vi "Write ZYState.vi"(7 "OPC UA AI list":string[](array[string]), 8 "error in (no error)":errorcluster, 10 "HE_state":T1 {"Y"."Y_Set" format="%.2f"; "Y"."SP" step=0.01 format="%.2f"; "Y"."Y" format="%.2f"; "Y"."PV" step=0.01 format="%.2f"; "Y"."SP_Set" step=0.01 format="%.2f"}, 11 "OPC UA server refnum in":T12) -> (0 "error out":errorcluster, 3 "OPC UA server refnum out":T12)   [LabVIEW 2019, in "OPC addons.lvlib"]
uses:
  OPC addons.lvlib
  <vilib>/OPCUA/controls/OPC UA Server Refnum.ctl
  Heating/ctl/ZYs_state_short.ctl
  Heating/ctl/ZY_state_short.ctl
  Heating/ctl/Z.ctl
  Heating/ctl/Z_source.ctl
  Heating/ctl/Z_State.ctl
  Heating/ctl/ZM_State.ctl
  Heating/ctl/Y_short.ctl
  Heating/ctl/Y_source.ctl
  Heating/ctl/Y_state.ctl
  Inputs/Ctl/Parameter State short.ctl
  Alarms/Ctl/ALR_Status_short.ctl
  Heating/ctl/ZY_state_OPC.ctl
  <vilib>/OPCUA/controls/Write Status.ctl
  <vilib>/OPCUA/server/Write Variant.vi
  <vilib>/OPCUA/NI OPC UA Server.lvlib
  Heating/Heating.lvlib
  Inputs/Inputs.lvlib
  Alarms/Alarms.lvlib
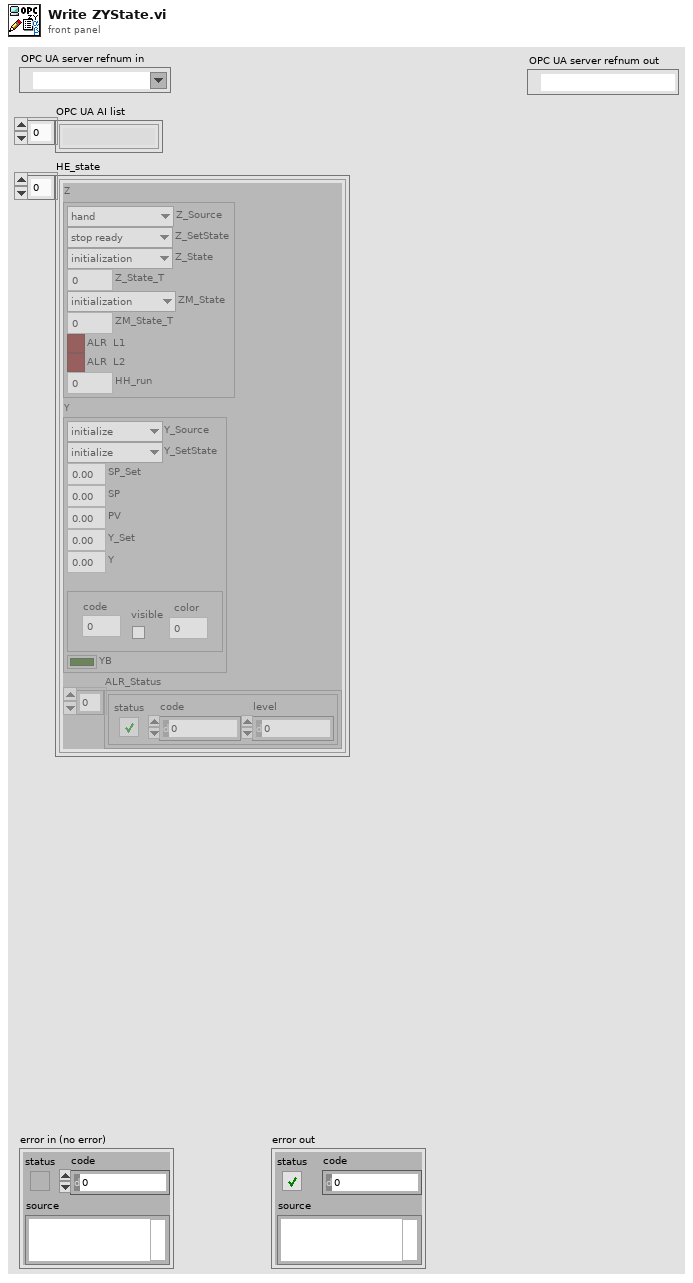
[diagram p1: front panel]
types:
  T1 = typedef "Heating.lvlib/ZYs_state_short.ctl" = T2[]
  T2 = typedef "Heating.lvlib/ZY_state_short.ctl" = cluster{"Z":T3, "Y":T7, "ALR_Status":T11[]}
  T3 = typedef "Heating.lvlib/Z.ctl" = cluster{"Z_Source":T4, "Z_SetState":T5, "Z_State":T5, "Z_State_T":u32, "ZM_State":T6, "ZM_State_T":u32, "ALR  L1":bool, "ALR  L2":bool, "HH_run":u64}
  T4 = typedef "Heating.lvlib/Z_source.ctl" = enum8{"initialize", "local disabled", "local hand", "hand", "auto", "dist"}
  T5 = typedef "Heating.lvlib/Z_State.ctl" = enum8{"initialization", "alarm", "disabled", "not ready", "stop ready", "reserv", "switched off", "reserv2", "switched on", "check", "on min", "decrease out", "on", "increase out", "on max"}
  T6 = typedef "Heating.lvlib/ZM_State.ctl" = enum8{"initialization", "stop", "start_cmd", "contactor_on_cmd", "heating", "on", "stop_cmd", "power_down", "contactor_off_cmd", "cooling", "restart_delay"}
  T7 = typedef "Heating.lvlib/Y_short.ctl" = cluster{"Y_Source":T8, "Y_SetState":T9, "SP_Set":dbl, "SP":dbl, "PV":dbl, "Y_Set":dbl, "Y":dbl, "Y_State":T10, "YB":bool}
  T8 = typedef "Heating.lvlib/Y_source.ctl" = enum8{"initialize", "local disabled", "local hand", "hand", "auto", "dist"}
  T9 = typedef "Heating.lvlib/Y_state.ctl" = enum8{"initialize", "alarm", "min", "stop", "hand", "auto", "max"}
  T10 = typedef "Inputs.lvlib/Parameter State short.ctl" = cluster{"code":i32, "visible":bool, "color":u32}
  T11 = typedef "Alarms.lvlib/ALR_Status_short.ctl" = cluster{"status":bool, "code":i32, "level":i32}
  T12 = typedef "OPC UA Server Refnum.ctl" = refnum<k21>
  T13 = typedef "Heating.lvlib/ZY_state_OPC.ctl" = cluster{"Z":cluster{"Z_Source":u8, "Z_SetState":u8, "Z_State":u8, "Z_State_T":u32, "ZM_State":u8, "ZM_State_T":u32, "ALR  L1":bool, "ALR  L2":bool, "HH_run":i32}, "Y":cluster{"Y_Source":u8, "Y_SetState":u8, "SP_Set":dbl, "SP":dbl, "PV":dbl, "Y_Set":dbl, "Y":dbl, "Y_State":cluster{"code":i32, "visible":bool, "color":u32}, "YB":bool}, "ALR_Status":cluster{"status":bool, "code":i32, "level":i32}[]}
  T14 = typedef "Write Status.ctl" = u32
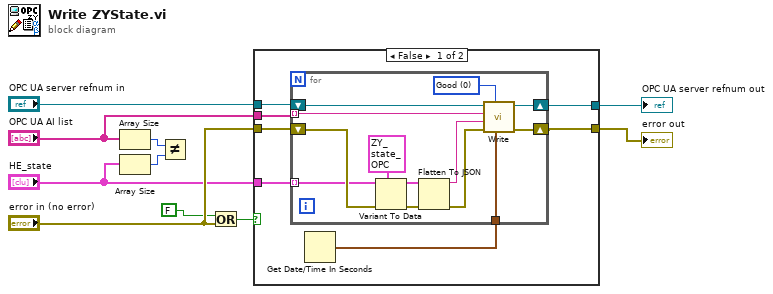
[diagram p0: block diagram]
diagram:
  n1 = Array Size(array="OPC UA AI list") -> (size(s)=w4:i32)
  n2 = Array Size(array="HE_state") -> (size(s)=w3:i32)
  n3 = Not Equal?(x=w4, y=w3) -> ()  [unwired: 1 out]
  n4 = Or(x=FALSE ("x != y?"), y="error in (no error)") -> (x .or. y?=w6:bool)
  n5 = case shown="False" w6 {
    tunnel: "OPC UA server refnum in" -> [w14 w32]
    tunnel: [w16 w32] -> w9
    tunnel: [w15 w31] -> w8
    tunnel: "OPC UA AI list" -> [w13 _]
    tunnel: "error in (no error)" -> [w12 w31]
    tunnel: "HE_state" -> [w11 _]
    frame False {
      n6 = Get Date/Time In Seconds() -> (seconds since 1Jan1904=w17:timestamp)
      n7 = for {
        tunnel: w17 -> [w29]
        tunnel: w13 -> [w28] mode=indexing
        shift-right: [w26] -> w16
        shift-left: w14 -> [w30]
        shift-right: [w25] -> w15
        shift-left: w12 -> [w20]
        tunnel: w11 -> [w19] mode=indexing
        w24 = T14 0 items=["Good"=0, "Uncertain"=1073741824, "Uncertain_InitialValue"=1083310080, "Uncertain_LastUsableValue"=1083179008, "Uncertain_SensorNotAccurate"=1083375616, "Uncertain_EngineeringUnitsExceeded"=1083441152, "Bad"=2147483648, "Bad_NoCommunication"=2150694912, "Bad_NotReadable"=2151284736, "Bad_NotWritable"=2151350272, "Bad_OutOfRange"=2151415808, "Bad_WaitingForInitialData"=2150760448] ("node status")
        n8 = Variant To Data(error in=w20, type=T13 {"Z"={"Z_Source"=0, "Z_SetState"=0, "Z_State"=0, "Z_State_T"=0, "ZM_State"=0, "ZM_State_T"=0, "ALR  L1"=FALSE, "ALR  L2"=FALSE, "HH_run"=0}, "Y"={"Y_Source"=0, "Y_SetState"=0, "SP_Set"=0.0, "SP"=0.0, "PV"=0.0, "Y_Set"=0.0, "Y"=0.0, "Y_State"={"code"=0, "visible"=FALSE, "color"=0}, "YB"=FALSE}, "ALR_Status"=[]} ("ZY_State"), Variant=w19) -> (data=w22:T13, error out=w21:errorcluster)
        n9 = Flatten To JSON(anything=w22, error in (no error)=w21) -> (JSON string=w27:string, 11:w23:errorcluster)  [unwired: 1 in]
        n10 = call-poly <vilib>:"Write.vi"("timestamp (current time)"=w29, "node status"=w24, "error in (no error)"=w23, "value"=w27, "node ID"=w28, "OPC UA server refnum in"=w30) -> ("error out"=w25:errorcluster, "OPC UA server refnum out"=w26:T12)  [unwired: 3 in, 1 out]
      }
    }
    frame True {
    }
  }
  "OPC UA server refnum out" <- w9
  "error out" <- w8
